vi "SavGlobalParams.vi"(7 "Task":enum16{"read", "write"}(ring), 9 "Color choices":T1={"Quote"=46086, "Comment"=15665920, "Python"=14453248, "Text"=0, "Triple Quote"=9306312, "function"=239, "Line numbers"=9306312, "REPL Err"=15665920, "REPL Text"=0, "Text Bkgd"=16777215, "REPL Bkgd"=16777215}, 11 "FileName":string="Colors.txt") -> (1 "Colors Out":T1={"Quote"=46086, "Comment"=15665920, "Python"=14453248, "Text"=0, "Triple Quote"=9306312, "function"=239, "Line numbers"=9306312, "REPL Err"=15665920, "REPL Text"=0, "Text Bkgd"=16777215, "REPL Bkgd"=16777215})   [LabVIEW 2020]
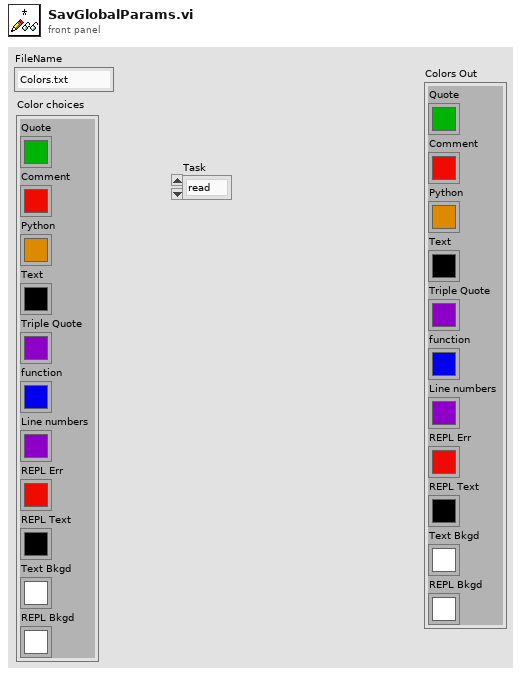
[diagram p1: front panel]
types:
  T1 = cluster{"Quote":u32, "Comment":u32, "Python":u32, "Text":u32, "Triple Quote":u32, "function":u32, "Line numbers":u32, "REPL Err":u32, "REPL Text":u32, "Text Bkgd":u32, "REPL Bkgd":u32}
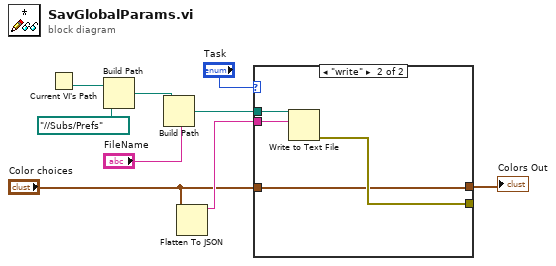
[diagram p0: block diagram]
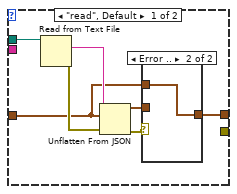
[diagram p2: hidden frame]
diagram:
  n1 = Current VI's Path() -> (path=w9:path)
  n2 = Build Path(base path=w9, name or relative path=path "../../Subs/Prefs") -> (appended path=w7:path)
  n3 = Build Path(base path=w7, name or relative path="FileName") -> (appended path=w5:path)
  n4 = Flatten To JSON(anything="Color choices") -> (JSON string=w4:string)  [unwired: 2 in, 1 out]
  n5 = case shown="\"write\"" "Task" {
    tunnel: w5 -> [w16 w22]
    tunnel: [_ w21] -> _
    tunnel: w4 -> [_ w20]
    tunnel: "Color choices" -> [w10 w19]
    tunnel: [w12 w19] -> w1
    frame "read", Default {
      n6 = Read from Text File(file (use dialog)=w16) -> (text=w15:string, error out=w14:errorcluster)  [unwired: 3 in, 2 out]
      n7 = Unflatten From JSON(JSON string=w15, type and defaults=w10, error in (no error)=w14) -> (value=w11:T1, error out=w13:errorcluster)  [unwired: 4 in]
      n8 = case shown="Error .." w13 {
        tunnel: [w17 w18] -> w12
        tunnel: w11 -> [w17 _]
        tunnel: w10 -> [_ w18]
        frame No Error {
        }
        frame Error {
        }
      }
    }
    frame "write" {
      n9 = Write to Text File(file (use dialog)=w22, text=w20) -> (error out=w21:errorcluster)  [unwired: 2 in, 2 out]
    }
  }
  "Colors Out" <- w1
